vi "Volt Regulator.vi"() -> ()   [LabVIEW 2014]
panel:
  in  "Volt High Threshold":dbl(slide)=6.5 scale=0.0..14.0
  in  "stop":bool
  out "NewGear":enum16{"High", "Low"}(ring)=enum."Low"
  in  "Volt Low Threshold":dbl(slide)=6.5 scale=0.0..14.0
  in  "HiEnabled":bool=TRUE
  in  "InVoltage":dbl(slide) scale=0.0..14.0
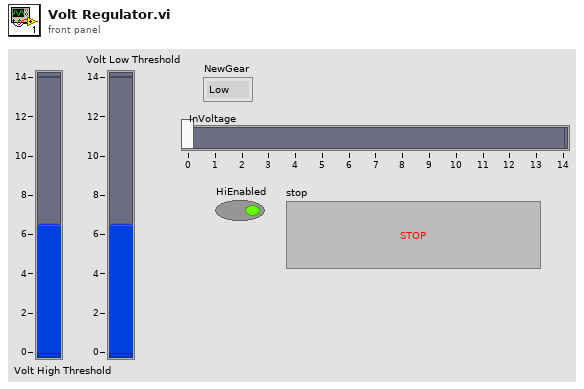
[diagram p1: front panel]
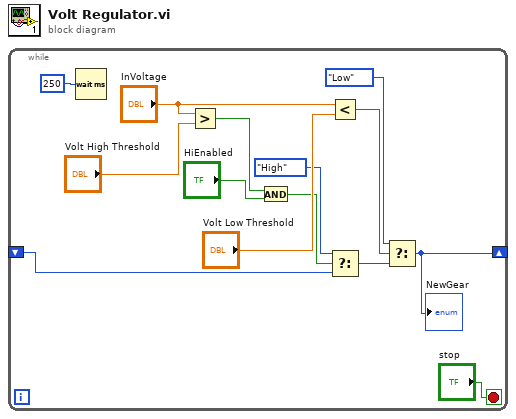
[diagram p0: block diagram]
diagram:
  n1 = while {
    shift-right: [w8] -> _
    shift-left: _ -> [w10]
    stop <- "stop" stop-if-true
    n2 = Wait (ms)(milliseconds to wait=u32 250) -> ()  [unwired: 1 out]
    n3 = Greater?(x="InVoltage", y="Volt High Threshold") -> (0:w3:bool)
    n4 = And(x=w3, y="HiEnabled") -> (x .and. y?=w1:bool)
    n5 = Less?(x="InVoltage", y="Volt Low Threshold") -> (x < y?=w14:bool)
    n6 = Select(t=enum16{"High", "Low"}."High" ("Gear 2"), s=w1, f=w10) -> (s? t:f=w9:enum16{"High", "Low"})
    n7 = Select(t=enum16{"High", "Low"}."Low" ("Gear 2"), s=w14, f=w9) -> (s? t:f=w8:enum16{"High", "Low"})
    "NewGear" <- w8
  }
